vi "Black Board Performance Test.vi"() -> ()   [LabVIEW 2021]
uses:
  Source/Blackboard/Blackboard.lvclass
  <vilib>/TSA/Abstract Data Classes/Abs_Types/Boolean/Static Read.vi
  Source/Blackboard/Support/Bool/Blackboard_Boolean.lvclass
  C:/Program Files (x86)/National Instruments/LabVIEW 2021/vi.lib/TSA/Abstract Data Classes/Abs_Types/Boolean/Abs_Boolean.lvclass
  <vilib>/TSA/Abstract Data Classes/Abs_Types/Boolean/Abs_Boolean.lvclass
  C:/Program Files (x86)/National Instruments/LabVIEW 2021/vi.lib/TSA/Abstract Data Classes/Abs_Types/Value/Abs_Value.lvclass
  C:/Program Files (x86)/National Instruments/LabVIEW 2021/vi.lib/TSA/Abstract Data Classes/Abs_Types/Type/Abs_Type.lvclass
  C:/Users/Tim/Documents/GitHub/LV_Behaviour_Tree/Source/Blackboard/Support/Bool/Blackboard_Boolean.lvclass
panel:
  out "x/y":dbl format="%#_6p"
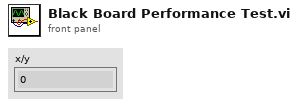
[diagram p1: front panel]
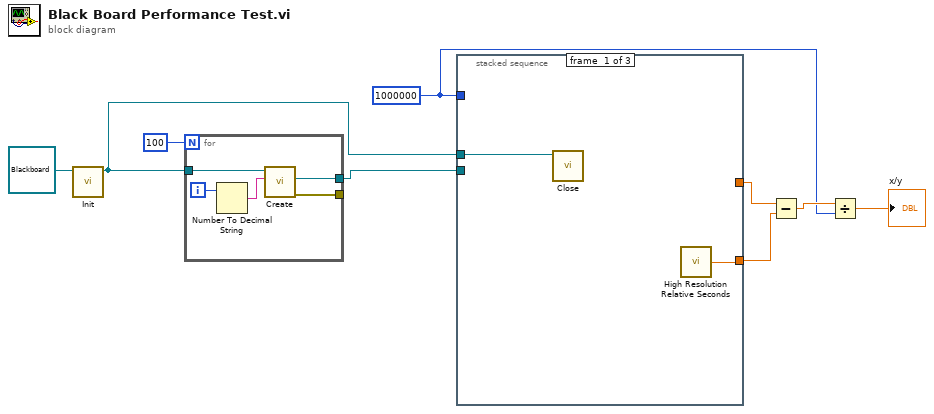
[diagram p0: block diagram]
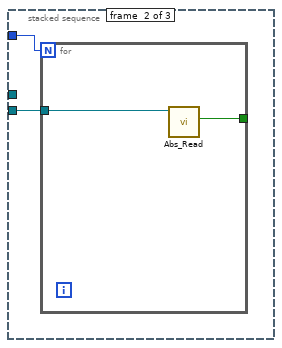
[diagram p2: hidden frame]
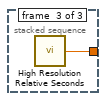
[diagram p3: hidden frame]
diagram:
  w3 = 1000000
  n1 = call-dynamic "Init.vi"("bt_Blackboard in"=refnum<class "Blackboard.lvclass"> refnum) -> ("bt_Blackboard out"=w1:refnum<class "Blackboard.lvclass">)  [unwired: 9 in, 1 out]
  n2 = for {
    N: 100 -> [_]
    tunnel: w1 -> [w14]
    tunnel: [w11] -> w8
    tunnel: [w10] -> _
    i -> [w12]
    n3 = Number To Decimal String(number=w12) -> (decimal integer string=w13:string)  [unwired: 1 in]
    n4 = call "Create.vi"("Tag"=w13, "Blackboard"=w14) -> ("error out"=w10:errorcluster, "Blackboard_Boolean.lvclass"=w11:refnum<class "Blackboard_Boolean.lvclass">)  [unwired: 7 in, 1 out]
  }
  n5 = stacked-sequence {
    tunnel: w8 -> [_ w18 _]
    tunnel: [w16 _ _] -> w5
    tunnel: [_ _ w21] -> w6
    tunnel: w3 -> [_ w17 _]
    tunnel: w1 -> [w15 _ _]
    frame #0 {
      n6 = call-dynamic "Close.vi"("bt_Blackboard in"=w15) -> ()  [unwired: 9 in, 2 out]
      n7 = call <vilib>:"High Resolution Relative Seconds.vi"() -> ("relative seconds"=w16:dbl)
    }
    frame #1 {
      n8 = for {
        N: w17 -> [_]
        tunnel: w18 -> [w19]
        tunnel: [w20] -> _
        n9 = call-poly <vilib>:"Abs_Read.vi"("Abs_Boolean in"=w19) -> ("Boolean"=w20:bool)  [unwired: 8 in, 2 out]
      }
    }
    frame #2 {
      n10 = call <vilib>:"High Resolution Relative Seconds.vi"() -> ("relative seconds"=w21:dbl)
    }
  }
  n11 = Subtract(x=w6, y=w5) -> (x-y=w4:dbl)
  n12 = Divide(x=w4, y=w3) -> (x/y=→"x/y":dbl)
